vi "SVI_ReadFromArduino.vi"(8 "error in (no error)":errorcluster, 11 "VISA Refnum in":refnum<visa-resource-name>) -> (0 "error out":errorcluster, 1 "Voltages":u16[](array[numeric]), 2 "Channels":u8[](array[numeric]), 3 "VISA Refnum out":refnum<visa-resource-name>)   [LabVIEW 2020]
panel:
  out "read buffer 2":string
  out "return count":u32
  out "Serial Settings:Number of Bytes at Serial Port":u32
  out "read buffer":string
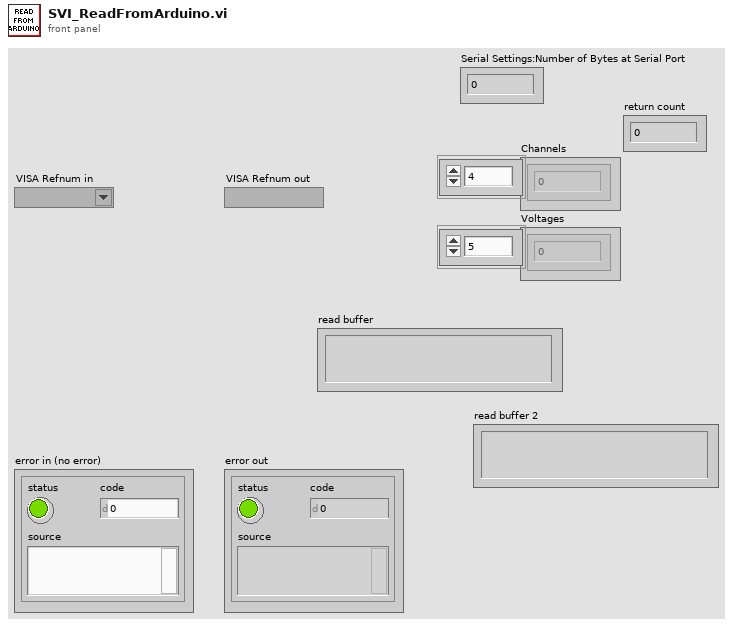
[diagram p1: front panel]
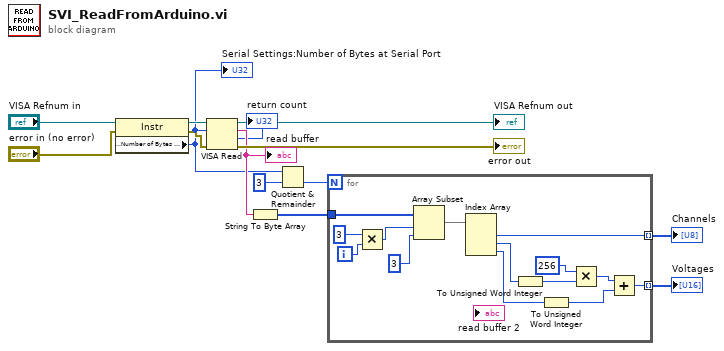
[diagram p0: block diagram]
diagram:
  n1 = property class="Instr"(reference="VISA Refnum in", error in="error in (no error)") -> (reference out=w6:refnum<visa-resource-name>, error out=w7:errorcluster, "Serial Settings:Number of Bytes at Serial Port"=w4:u32)
  "Serial Settings:Number of Bytes at Serial Port" <- w4
  n2 = VISA Read(VISA resource name=w6, byte count=w4, error in (no error)=w7) -> (VISA resource name out=→"VISA Refnum out":refnum<visa-resource-name>, read buffer=w5:string, return count=→"return count":u32, error out=→"error out":errorcluster)
  "read buffer" <- w5
  n3 = String To Byte Array(string=w5) -> (unsigned byte array=w12:u8[])
  n4 = Quotient & Remainder(x=w4, y=u32 3) -> (floor(x/y)=w2:u32)  [unwired: 1 out]
  n5 = for {
    N: w2 -> [_]
    tunnel: w12 -> [w26]
    tunnel: [w16] -> w11 mode=indexing
    tunnel: [w15] -> w10 mode=indexing
    i -> [w28]
    n6 = Multiply(x=3, y=w28) -> (x*y=w25:i32)
    n7 = Array Subset(array=w26, index=w25, length=3) -> (w17:u8[])
    n8 = Index Array(array=w17) -> (element #1=w16:u8, element #2=w23:u8, element #3=w20:u8)  [unwired: 3 in]
    n9 = To Unsigned Word Integer(number=w23) -> (unsigned 16bit integer=w19:u16)
    n10 = To Unsigned Word Integer(number=w20) -> (unsigned 16bit integer=w18:u16)
    n11 = Multiply(x=u16 256, y=w19) -> (x*y=w21:u16)
    n12 = Add(x=w21, y=w18) -> (x+y=w15:u16)
  }
  "Channels" <- w11
  "Voltages" <- w10
